vi "Add To Grid.vi"(1 "Object Index in":i16, 2 "Simulation Object in":refnum<class "SimulationObject.lvclass">, 3 "Collision Grid in":refnum<class "CollisionGrid.lvclass">) -> (0 "Collision Grid out":refnum<class "CollisionGrid.lvclass">)   [LabVIEW 2022 SP3, in "CollisionGrid.lvclass"]
uses:
  CollisionGrid.lvclass
  SimulationObject/SimulationObject.lvclass
  SimulationObject/SimulationObject.lvclass/SimulationObject.ctl
  Components/Transform/Transform.lvclass/Transform.ctl
  CollisionGrid.lvclass/CollisionGrid.ctl
  Math/Vector2/Vector2.lvclass/Vector2.ctl
  Math/Vector2/Read x.vi
  Math/Vector2/Read y.vi
  Components/Transform/Transform.lvclass
  Math/Vector2/Vector2.lvclass
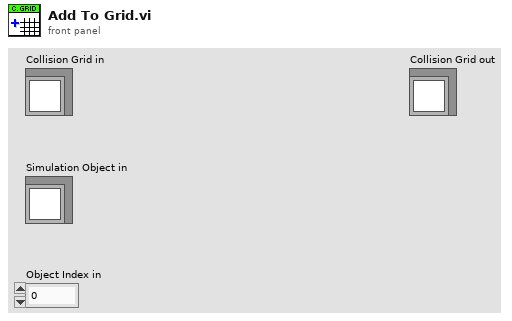
[diagram p1: front panel]
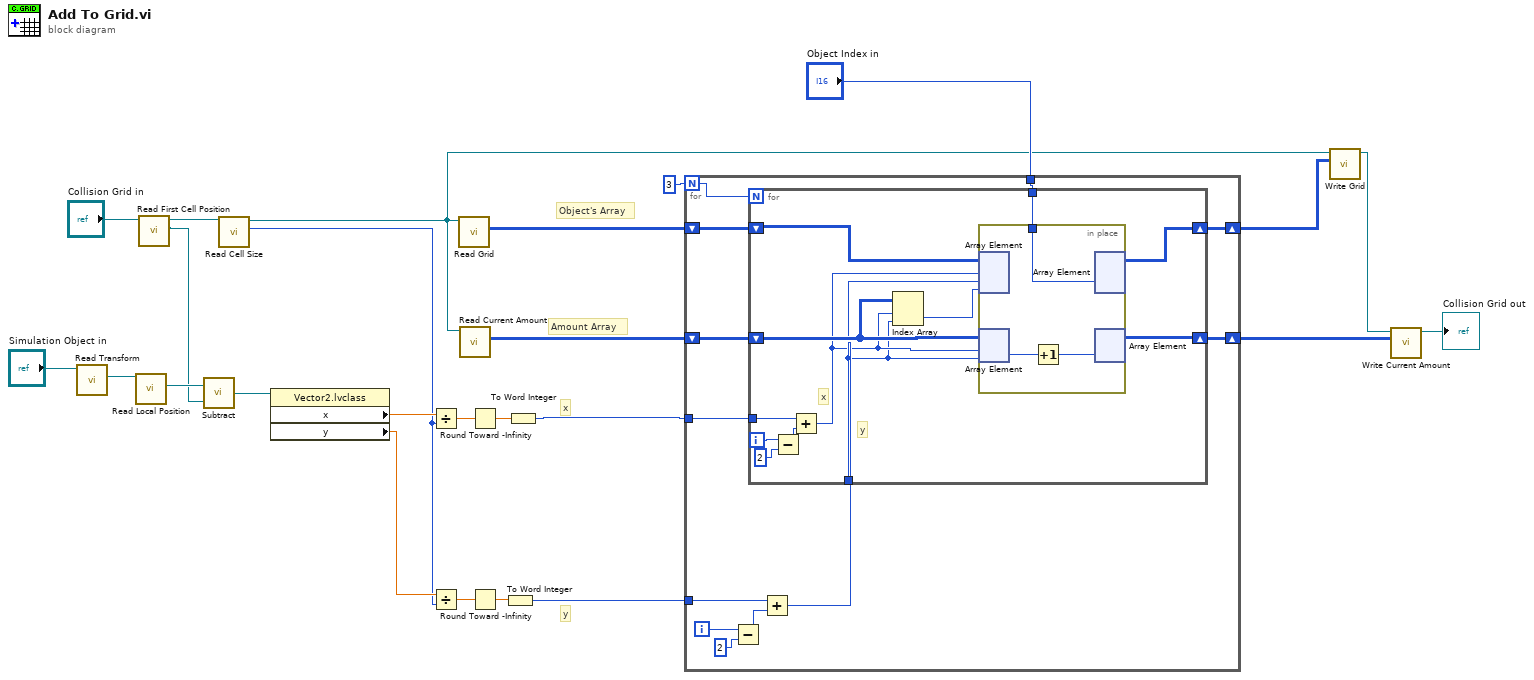
[diagram p0: block diagram]
diagram:
  # "Object's Array"
  # "Amount Array"
  # "y"
  # "x"
  n1 = call "Read Transform.vi"("SimulationObject in"="Simulation Object in") -> ("Transform out"=w24:refnum<class "Transform.lvclass">)  [unwired: 8 in, 2 out]
  n2 = call "Read Local Position.vi"("Transform in"=w24) -> ("Local Position out"=w22:refnum<class "Vector2.lvclass">)  [unwired: 8 in, 2 out]
  n3 = call "Read First Cell Position.vi"("CollisionGrid in"="Collision Grid in") -> ("First Cell Position out"=w21:refnum<class "Vector2.lvclass">, "CollisionGrid out"=w19:refnum<class "CollisionGrid.lvclass">)  [unwired: 8 in, 1 out]
  n4 = call "Subtract.vi"("Vec2 b in"=w21, "Vec2 a in"=w22) -> ("Vec2 out"=w20:refnum<class "Vector2.lvclass">)
  n5 = call "Read Cell Size.vi"("CollisionGrid in"=w19) -> ("Cell Size"=w16:i16, "CollisionGrid out"=w4:refnum<class "CollisionGrid.lvclass">)  [unwired: 8 in, 1 out]
  n6 = property class="Vector2.lvclass"(reference=w20) -> ("x"=w18:sgl, "y"=w17:sgl)  [unwired: 1 in, 2 out]
  n7 = Divide(x=w18, y=w16) -> (x/y=w15:sgl)
  n8 = Divide(x=w17, y=w16) -> (x/y=w14:sgl)
  n9 = call "Read Grid.vi"("CollisionGrid in"=w4) -> ("Grid"=w8:i16[][][])  [unwired: 8 in, 2 out]
  n10 = call "Read Current Amount.vi"("CollisionGrid in"=w4) -> ("Current Amount"=w5:i16[][])  [unwired: 8 in, 2 out]
  n11 = Round Toward -Infinity(1:w15) -> (0:w10:sgl)
  n12 = Round Toward -Infinity(1:w14) -> (0:w12:sgl)
  n13 = To Word Integer(number=w12) -> (16bit integer=w11:i16)
  n14 = To Word Integer(number=w10) -> (16bit integer=w9:i16)
  n15 = for {
    N: 3 -> [w37]
    tunnel: w9 -> [w36]
    tunnel: w11 -> [w32]
    shift-right: [w30] -> w6
    shift-left: w8 -> [w31]
    tunnel: "Object Index in" -> [w28]
    shift-right: [w26] -> w3
    shift-left: w5 -> [w27]
    i -> [w35]
    n16 = Subtract(x=w35, y=i16 2) -> (x-y=w33:i32)
    n17 = Add(x=w32, y=w33) -> (x+y=w29:i32)
    n18 = for {
      N: w37 -> [_]
      tunnel: w36 -> [w46]
      shift-right: [w43] -> w30
      shift-left: w31 -> [w45]
      tunnel: w29 -> [w40]
      tunnel: w28 -> [w44]
      shift-right: [w38] -> w26
      shift-left: w27 -> [w42]
      i -> [w48]
      # "y"
      # "x"
      n19 = Subtract(x=w48, y=i16 2) -> (x-y=w47:i32)
      n20 = Add(x=w46, y=w47) -> (x+y=w41:i32)
      n21 = Index Array(array=w42, index (row)=w41, index (col)=w40) -> (element=w39:i16)
      n22 = in-place {
        in-place-border: w44 -> [w52]
        n23 = in-place-array #1(w45, w41, w40, w39) -> ()  [unwired: 1 out]
        n24 = in-place-array #2(w42, w41, w40) -> (w51:i16)
        n25 = Increment(x=w51) -> (x+1=w50:i16)
        n26 = in-place-array #1(w52) -> (w43:i16[][][])  [unwired: 3 out]
        n27 = in-place-array #2(w50) -> (w38:i16[][])  [unwired: 2 out]
      }
    }
  }
  n28 = call "Write Grid.vi"("Grid"=w6, "CollisionGrid in"=w4) -> ("CollisionGrid out"=w2:refnum<class "CollisionGrid.lvclass">)  [unwired: 8 in, 1 out]
  n29 = call "Write Current Amount.vi"("Current Amount"=w3, "CollisionGrid in"=w2) -> ("CollisionGrid out"=→"Collision Grid out":refnum<class "CollisionGrid.lvclass">)  [unwired: 8 in, 1 out]
